vi "2.1.vi"() -> ()   [LabVIEW 2020]
panel:
  out "Actual":dbl
  out "Anterior":dbl
  out "i=":dbl
  in  "Numero de elementos en la serie Fibonacci":i32
  out "Array":dbl[](array[numeric])
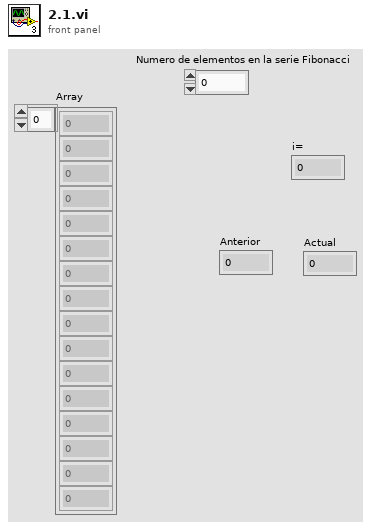
[diagram p1: front panel]
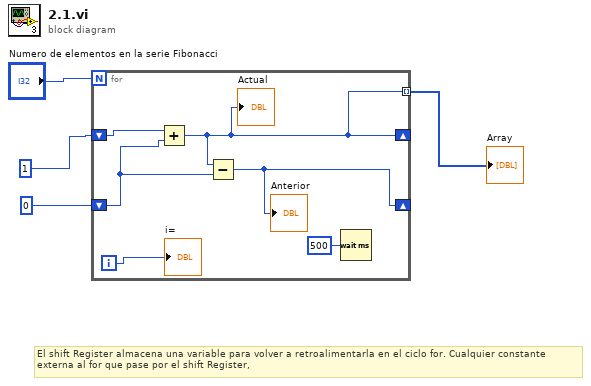
[diagram p0: block diagram]
diagram:
  # "El shift Register almacena una variable para volver a retroalimentarla en el ciclo for. Cualquier constante\nexterna al for que pase por el shift Register,"
  n1 = for {
    N: "Numero de elementos en la serie Fibonacci" -> [_]
    shift-right: [w5] -> _
    shift-left: 1 -> [w7]
    shift-right: [w6] -> _
    shift-left: 0 -> [w8]
    tunnel: [w5] -> w1 mode=indexing
    i -> [w9]
    n2 = Add(x=w7, y=w8) -> (x+y=w5:i32)
    "Actual" <- w5
    n3 = Subtract(x=w5, y=w8) -> (x-y=w6:i32)
    "Anterior" <- w6
    n4 = Wait (ms)(milliseconds to wait=u32 500) -> ()  [unwired: 1 out]
    "i=" <- w9
  }
  "Array" <- w1
